vi "PvgeneratorOP300.2.vi"(8 "errin":errorcluster, 10 "network":path, 11 "path in":path) -> (0 "sortie d'erreur":errorcluster caption="errout", 1 "network out":path, 2 "tout bon":bool, 3 "Chaîne":string)   [LabVIEW 2020]
uses:
  VG/IS30%.vi
  VG/PN.vi
  <vilib>/Utility/config.llb/NI_LVConfig.lvlib
  SubVI/VG_HYDRAU.vi
panel:
  out "nombre de remplacements":i32
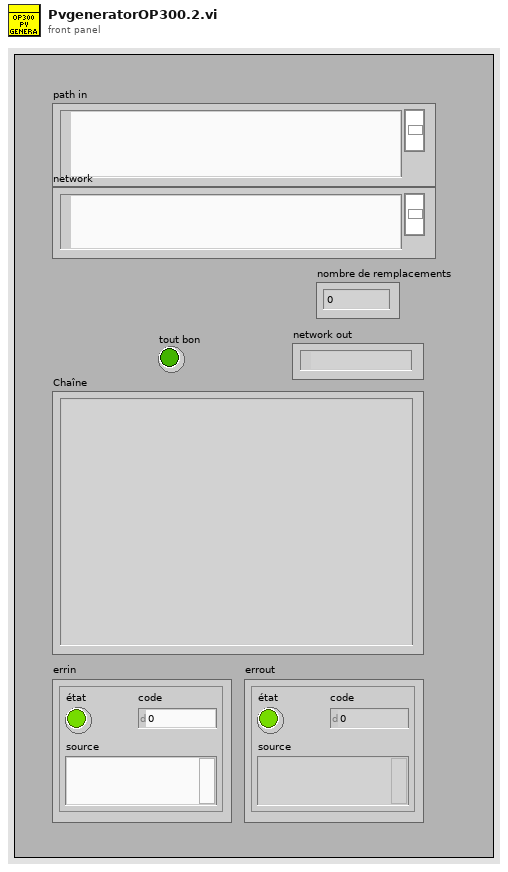
[diagram p1: front panel]
types:
  T1 = enum16{"open", "replace", "create", "open or create", "replace or create", "replace or create with confirmation"}
  T2 = typedef "NI_LVConfig.lvlib/Config Data RefNum.ctl" = refnum<k1>
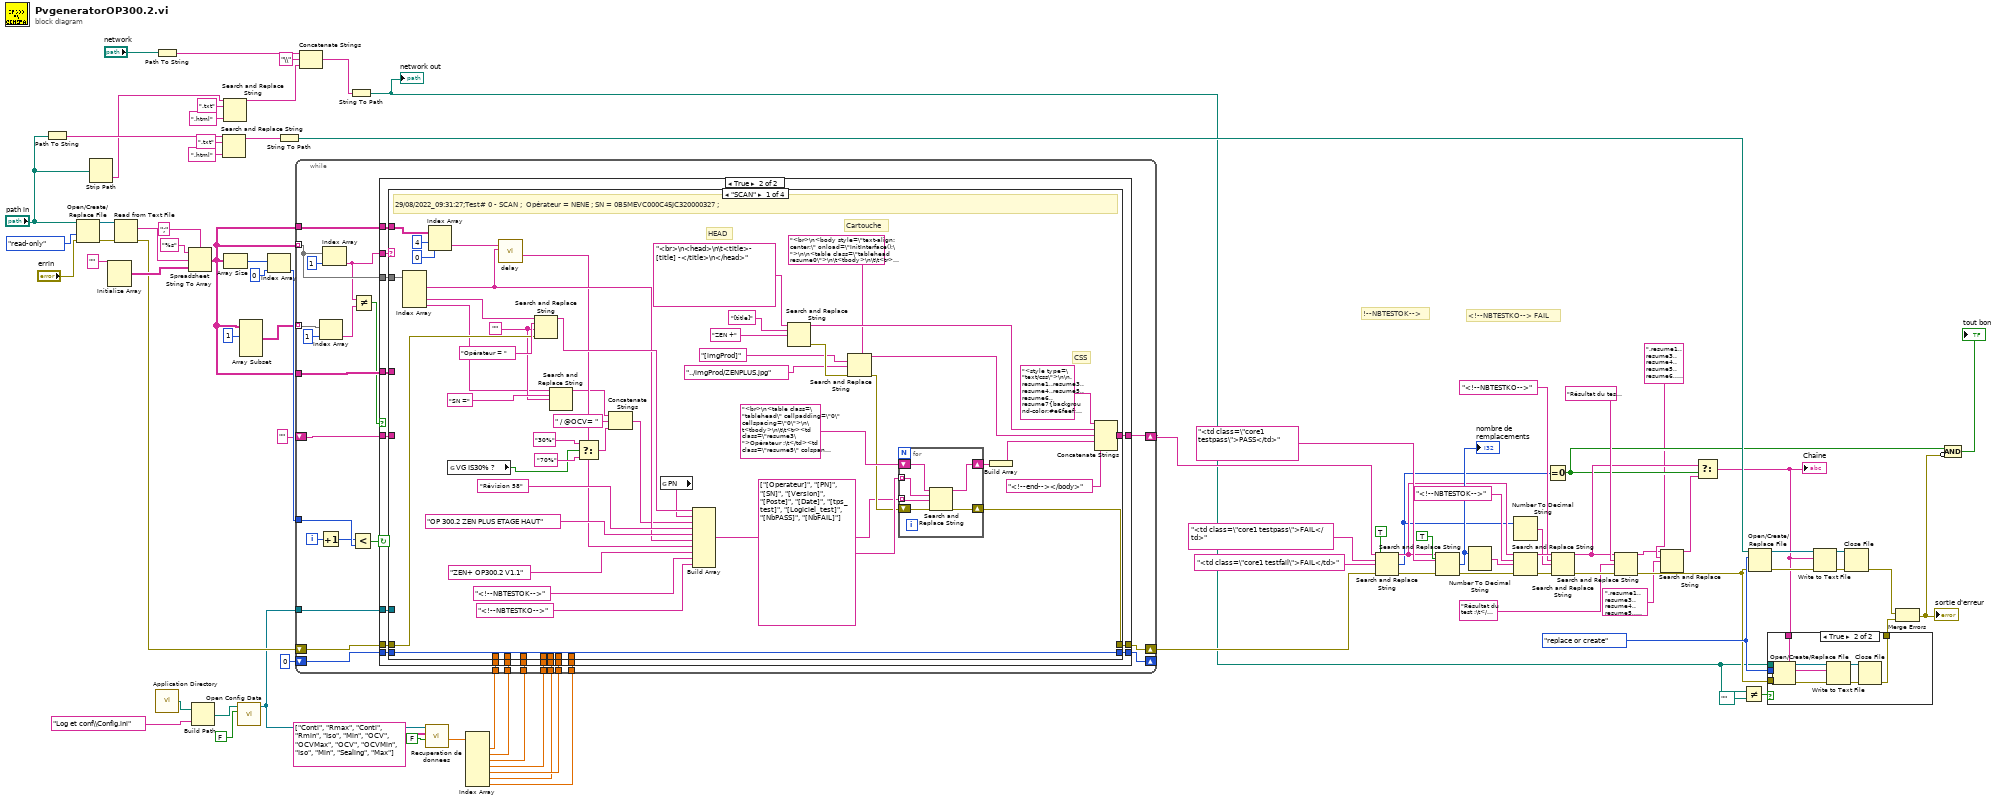
[diagram p0: block diagram]
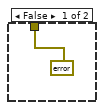
[diagram p2: hidden frame]
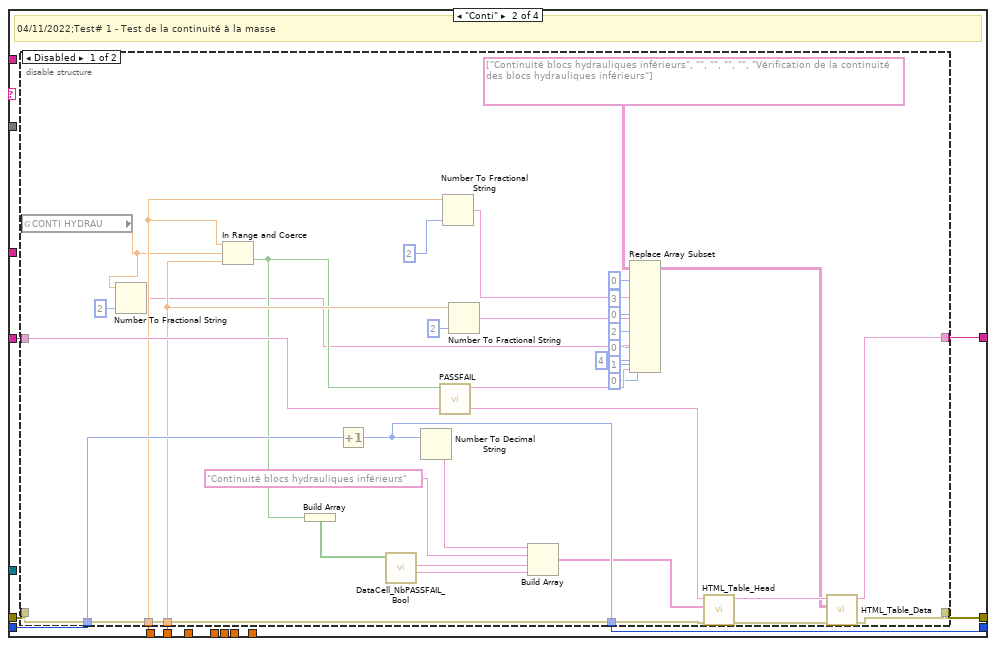
[diagram p4: hidden frame]
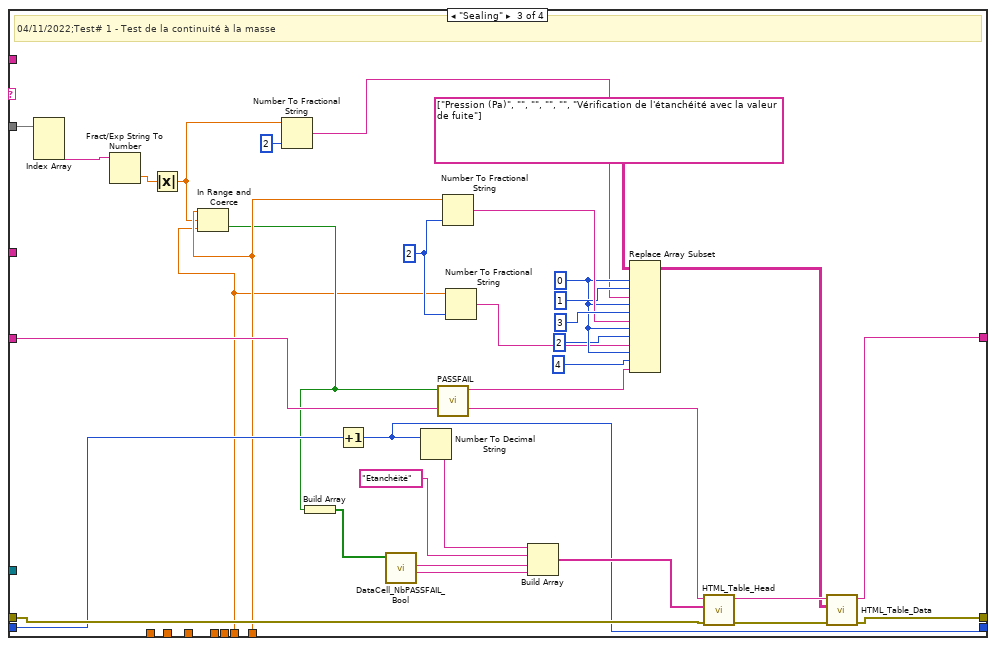
[diagram p6: hidden frame]
diagram:
  w47 = T1."replace or create" ("opération (0 : open)")
  # "<!--NBTESTKO--> FAIL"
  # "!--NBTESTOK-->"
  n1 = Path To String(path="path in") -> (string=w69:string)
  n2 = Open/Create/Replace File(file path (use dialog)="path in", error in="errin", access (0:read/write)=enum16{"read/write", "read-only", "write-only"}."read-only" ("accès (0 : read/write)")) -> (refnum out=w70:refnum<file>, error out=w87:errorcluster)  [unwired: 3 in, 1 out]
  n3 = Strip Path(path="path in") -> (name=w28:string)  [unwired: 1 out]
  n4 = Initialize Array("") -> (w85:string[][])  [unwired: 2 in]
  n5 = Read from Text File(file (use dialog)=w70, error in=w87) -> (text=w83:string, error out=w75:errorcluster)  [unwired: 2 in, 2 out]
  n6 = Path To String(path="network") -> (string=w27:string)
  n7 = call <vilib>:"Application Directory.vi"() -> ("Application Directory"=w19:path)
  n8 = Spreadsheet String To Array(delimiter (Tab)=";" ("séparateur (Tabulation)"), format string="%s" ("chaîne de format"), spreadsheet string=w83, array type (2D Dbl)=w85) -> (array=w6:string[][])
  n9 = Build Path(base path=w19, name or relative path="Log et conf\\Config.ini") -> (appended path=w22:path)
  n10 = Search and Replace String(input string=w69, search string=".txt" ("chaîne recherchée"), replace string=".html" ("chaîne de remplacement (\"\")")) -> (result string=w66:string)  [unwired: 5 in, 3 out]
  n11 = Search and Replace String(input string=w28, search string=".txt" ("chaîne recherchée"), replace string=".html" ("chaîne de remplacement (\"\")")) -> (result string=w25:string)  [unwired: 5 in, 3 out]
  n12 = Array Size(array=w6) -> (size(s)=w81:i32[])
  n13 = call <vilib>:"Open Config Data.vi"("create file if necessary (T)"=FALSE, "configuration file path"=w22) -> ("refnum"=w1:T2)  [unwired: 7 in, 2 out]
  n14 = Array Subset(array=w6, index (row)=1 ("indice")) -> (w4:string[][])  [unwired: 3 in]
  n15 = Index Array(array=w81, index=0 ("indice")) -> (element=w79:i32)
  n16 = String To Path(string=w66) -> (path=w65:path)
  n17 = Concatenate Strings(w27, "\\" ("chaîne"), w25) -> (w24:string)
  n18 = String To Path(string=w24) -> (path=w30:path)
  "network out" <- w30
  n19 = call "Recuperation de donnees.vi"("Est-ce un string?"=FALSE, "Array in"=string[][] [["Conti", "Rmax"], ["Conti", "Rmin"], ["Iso", "Min"], ["OCV", "OCVMax"], ["OCV", "OCVMin"], ["Iso", "Min"], ["Sealing", "Max"]], "Refnum in"=w1) -> ("Array"=w16:dbl[])  [unwired: 7 in, 1 out]
  n20 = Index Array(array=w16) -> (element #1=w15:dbl, element #2=w14:dbl, element #3=w13:dbl, element #4=w12:dbl, element #5=w11:dbl, element #6=w3:dbl, element #7=w2:dbl)  [unwired: 7 in]
  n21 = while {
    tunnel: w79 -> [w114]
    tunnel: w6 -> [w111] mode=indexing
    shift-right: [w110] -> w62
    shift-left: w75 -> [w109]
    shift-right: [w103] -> w64
    shift-left: "" -> [w108]
    shift-right: [w106] -> _
    shift-left: 0 -> [w107]
    tunnel: w6 -> [w105]
    tunnel: w15 -> [w102]
    tunnel: w14 -> [w101]
    tunnel: w6 -> [w100]
    tunnel: w13 -> [w99]
    tunnel: w12 -> [w98]
    tunnel: w11 -> [w97]
    tunnel: w4 -> [w95] mode=indexing
    tunnel: w3 -> [w91]
    tunnel: w2 -> [w90]
    tunnel: w1 -> [w89]
    i -> [w115]
    stop <- w113 continue-if-true
    n22 = Index Array(array=w95, index=1 ("indice")) -> (element=w94:string)
    n23 = Increment(x=w115) -> (x+1=w104:i32)
    n24 = Index Array(array=w111, index=1 ("indice")) -> (element=w93:string)
    n25 = Less?(x=w104, y=w114) -> (x < y?=w113:bool)
    n26 = Not Equal?(x=w93, y=w94) -> (x != y?=w92:bool)
    n27 = case shown="True" w92 {
      tunnel: w111 -> [_ w136]
      tunnel: [w117 w135] -> w110
      tunnel: w109 -> [w117 w134]
      tunnel: w108 -> [w118 w133]
      tunnel: w107 -> [w116 w132]
      tunnel: [w116 w131] -> w106
      tunnel: w105 -> [_ w130]
      tunnel: [w118 w129] -> w103
      tunnel: w93 -> [_ w128]
      tunnel: w102 -> [_ w127]
      tunnel: w101 -> [_ w126]
      tunnel: w100 -> [_ w125]
      tunnel: w99 -> [_ w124]
      tunnel: w98 -> [_ w123]
      tunnel: w97 -> [_ w122]
      tunnel: w91 -> [_ w121]
      tunnel: w90 -> [_ w120]
      tunnel: w89 -> [_ w119]
      frame False {
      }
      frame True {
        n28 = case shown="\"SCAN\"" w128 {
          tunnel: w134 -> [w181 w197 w259 w269]
          tunnel: w136 -> [w183 _ w260 _]
          tunnel: [w160 w196 w258 w269] -> w135
          tunnel: w133 -> [_ w195 w257 w267]
          tunnel: w132 -> [w159 w194 w256 w268]
          tunnel: [w159 w193 w255 w268] -> w131
          tunnel: w130 -> [_ _ _ _]
          tunnel: [w158 w192 w254 w267] -> w129
          tunnel: w127 -> [_ w191 _ _]
          tunnel: w126 -> [_ w190 _ _]
          tunnel: w125 -> [w151 _ _ _]
          tunnel: w124 -> [_ _ _ _]
          tunnel: w123 -> [_ _ _ _]
          tunnel: w122 -> [_ _ w238 _]
          tunnel: w121 -> [_ _ _ _]
          tunnel: w120 -> [_ _ w242 _]
          tunnel: w119 -> [_ _ _ _]
          frame "SCAN" {
            w154 = ""
            # "Cartouche"
            # "HEAD"
            # "CSS"
            # "29/08/2022_09:31:27;Test# 0 - SCAN ;  Opérateur = NENE ; SN = 0B5MEVC000C45JC320000327 ;"
            n29 = Index Array(array=w183) -> (element #1=w147:string, element #3=w157:string, element #4=w152:string)  [unwired: 4 in, 1 out]
            n30 = Index Array(array=w151, index (row)=4, index (col)=0 ("disabled index (col)")) -> (element=w148:string)
            n31 = global read "IS30%.vi" "VG IS30% ?"() -> (w138:bool)
            n32 = call "delay.vi"("String"=w147, "String 2"=w148) -> ("Delay calculé"=w146:string)  [unwired: 9 in]
            n33 = Search and Replace String(input string=w157, search string="Opérateur = " ("chaîne recherchée"), replace string=w154, error in=w181) -> (result string=w156:string)  [unwired: 4 in, 3 out]
            n34 = Search and Replace String(input string=w152, search string="SN =" ("chaîne recherchée"), replace string=w154) -> (result string=w144:string)  [unwired: 5 in, 3 out]
            n35 = Select(t="30%" ("y"), s=w138, f="70%" ("y")) -> (s? t:f=w141:string)
            n36 = Concatenate Strings(w144, " / @OCV= " ("chaîne"), w141) -> (w143:string)
            n37 = global read "PN.vi" "PN"() -> (w137:string)
            n38 = Build Array(w156, w137, w143, "Révision 58" ("element"), "OP 300.2 ZEN PLUS ETAGE HAUT" ("chaîne"), w147, w146, "ZEN+ OP300.2 V1.1" ("chaîne"), "<!--NBTESTOK-->" ("chaîne"), "<!--NBTESTKO-->" ("chaîne")) -> (w161:string[])
            n39 = Search and Replace String(input string="<br>\n<head>\n\t<title>- [title] -</title>\n</head>", search string="[title]" ("chaîne recherchée"), replace string="ZEN +" ("Title")) -> (result string=w177:string, error out=w176:errorcluster)  [unwired: 5 in, 2 out]
            n40 = Search and Replace String(input string="<br>\n<body style=\"text-align: center;\" onload=\"InitInterface();\">\n\n<table class=\"tablehead resume0\">\n\t<tbody>\n\t\t<tr>\n\t\t\t<td> <img src=\"[imgProd]\" style=\"width:194px;height:100px\" class=\"left\"></td>\n\t\t\t<td> <div class=\"center\">PROCES VERBAL DE TEST AUTOMATIQUE</div><div class=\"center\">Zen Plus OP 300.2</div><br class=\"center\"><div class=\"center\">Forseepower</div></td>\n\t\t\t<td> <img src=\"../imgProd/LOGO FORSEE.png\" style=\"width:auto;height:auto\"  class=\"right\"></td>\n\t\t</tr>\n\t</tbody>\n</table>", search string="[imgProd]", replace string="../imgProd/ZENPLUS.jpg" ("imgProd"), error in=w176) -> (result string=w174:string, error out=w171:errorcluster)  [unwired: 4 in, 2 out]
            n41 = for {
              shift-right: [w188] -> w170
              shift-left: "<br>\n<table class=\"tablehead\" cellpadding=\"0\" cellspacing=\"0\">\n\t<tbody>\n\t\t<tr><td class=\"resume3\">Opérateur :\t</td><td class=\"resume5\" colspan=\"3\">[Operateur]</td></tr>\n\t\t<tr><td class=\"resume3\">PN : </td><td class=\"resume5\" colspan=\"3\">[PN]</td></tr>\n\t\t<tr><td class=\"resume3\">SN : </td><td class=\"resume5\" colspan=\"3\">[SN]</td></tr>\n\t\t<tr><td class=\"resume3\">Version : </td><td class=\"resume5\" colspan=\"3\">[Version]</td></tr>\n\t\t<tr><td class=\"resume3\">Poste : </td><td class=\"resume5\" colspan=\"3\">[Poste]</td></tr>\t\t\n\t\t<tr><td class=\"resume3\">Date du test : </td><td class=\"resume5\" colspan=\"3\">[Date]</td></tr>\n\t\t<tr><td class=\"resume3\">Temps de test : </td><td class=\"resume5\" colspan=\"3\">[tps_test]</td></tr>\n\t\t<tr><td class=\"resume3\">Logiciel de test :\t</td><td class=\"resume5\" colspan=\"3\">[Logiciel_test]</td></tr>\n\t\t<tr><td class=\"resume3\">Résultat du test :\t</td><td class=\"resume5\" colspan=\"3\"><div><span style=\"float:left\" id=\"result\"><font size = \"5pt\" color=\"green\"><b>CONFORME</b></font><b><font size = \"5pt\"> ( </font><font size = \"5pt\" color=\"green\">[NbPASS] PASS </font>  <font size = \"5pt\"> / </font><font size = \"5pt\" color=\"red\">[NbFAIL] FAIL</font> <font size = \"5pt\"> ) </font></b></span></div></td></tr>\n\t</tbody>\n</table>" -> [w189]
              tunnel: string[] ["[Operateur]", "[PN]", "[SN]", "[Version]", "[Poste]", "[Date]", "[tps_test]", "[Logiciel_test]", "[NbPASS]", "[NbFAIL]"] -> [w185] mode=indexing
              tunnel: w161 -> [w184] mode=indexing
              shift-right: [w186] -> w160
              shift-left: w171 -> [w187]
              n42 = Search and Replace String(input string=w189, search string=w185, replace string=w184, error in=w187) -> (result string=w188:string, error out=w186:errorcluster)  [unwired: 4 in, 2 out]
            }
            n43 = Build Array(w170) -> (w169:string[])
            n44 = Concatenate Strings("<style type=\"text/css\">\n\n.resume1,.resume3,.resume4,.resume5,.resume6,.resume7{background-color:#e6feef;padding:7px;border:1px solid black;}\n.resume0{border:1px solid black;background-color:#e6feef;font-weight: bold;padding:0px;text-align: center;}\n.resume1{width:350px;text-align:right;font-weight:bold;}\n.resume3{width:350px;text-align:right;border-top:0px solid black;font-weight:bold;}\n.resume4{border-left:0px solid black;width:290px;}\n.resume5{width:290px;border-left:0px solid black;border-top:0px solid black;}\n.resume6{border-left:0px solid black;width:60px;}\n.resume7{border-left:0px solid black;border-top:0px solid black;width:60px;}\n.title1{text-align: left;background-color:#e6f4fe;padding:10px;border:1px solid #101010;}\n.title2{width: 30px;text-align: center;background-color:#e6f4fe;padding:1px;border:1px solid #101010;border-left:0px solid black;font-weight: bold;}\n.title2 a:link{text-decoration:none;}\n.entete0,.entete1,.entete2,.time2{text-align: center;background-color:#feeec9;padding:7px;border:1px solid black;font-weight: bold;}\n.entete0{width:45px;border-right:0px solid black;}\n.entete1{width:505px;}\n.entete2{width:95px;border-right:0px solid black;}\n.time2{border-left:0px solid black;width:145px;font-size:11px;}\n.core0,.core1,.core2,.core3,.core4,.time{text-align: center;background-color:#fafed3;padding:7px;border:1px solid black;}\n.core0, .core1,.core3,.core4{width:95px;border-top:0px solid black;border-right:0px solid black;}\n.core0{width:45px;}\n.core2{border-top:0px solid black;width:505px;}\n.core3{width:200px;}\n.core4{width:300px;}\n.time{width:145px;border-top:0px solid black;border-left:0px solid black;font-size:11px;}\n.false .core0,.false .core1,.false .core2,.false .core3,.false .core4,.false .time{background-color:#f4f4f4;}\n.false .entete0,.false .entete1,.false .entete2,.false .time2{background-color:#dadada;}\n.false .title1,.false .title2,.false .resultentete .testpass,.false .resultentete .testfail,.false .resultentete .testtime{background-color:#c5cac9;color: blue;}\n.false .title2 a:link{text-decoration:none;color: blue;}\n.comment1,.comment2,.time3{width: 890px;background-color:#e9e8e9;padding:7px;border:1px solid black;border-top:0px solid black;text-align:left;}\n.comment2{border-right:0px solid black;width: 45px;text-align: center;}\n.time3{width: 145px;border-left:0px solid black;font-size:11px;}\n.fixe1{background: -moz-linear-gradient(center top , #101010 10%, #555555 80%) repeat scroll 0 0 transparent;background: -webkit-gradient(linear, left top, left bottom, from(#101010), to(#555555));border:2px solid orange;position : fixed;margin-top:20px;display:none;overflow-y:scroll;max-height:350px;text-shadow: 0px 0px 0 #333333;text-align:left;font-size:10px;padding:10px;margin-left:-162px;border-radius: 15px 15px 15px 15px;}\n.menufixe, .menufixelock{background: -moz-linear-gradient(center top , #101010 80%, transparent 20%) repeat scroll 0 0 transparent;background: -webkit-gradient(linear, left top, left bottom, from(#101010), color-stop(0.65, #101010), to(transparent)) repeat scroll 0 0 transparent;margin: -52px 0px 0px -9px;width:100%;position:fixed;height:55px;-moz-transition: margin 1s;-webkit-transition: margin 1s;}\n.menufixelock, .menufixe:hover{margin: -9px 0px 0px -9px;}\n.lockmenu, .separation,.separationmenu{text-align:center;background: -moz-linear-gradient(center top , #555555 10%, #111111 80%) repeat scroll 0 0 transparent;background: -webkit-gradient(linear, left top, left bottom, from(#555555), to(#111111));border: 1px solid white;border-radius: 10px 10px 10px 10px;box-shadow: 0 -1px 1px #555555 inset;color: #999999;font-weight: bold;width: 100px;padding: 2px;text-decoration: none;}\n.tablehead{width: 1000px;font-family: Verdana;font-size: 12px;margin-left: auto;margin-right: auto;}\n.tablenull{font-family: Verdana;font-size: 11px;margin-left: auto;margin-right: auto;}\n.separationmenu:hover div{display: inline;}\n.lockmenu:hover, .separation:hover,.separationmenu:hover{border: 1px solid orange;cursor:pointer;}\n.lockmenu:hover{border: 1px solid red;cursor:pointer;}\n.separationright{padding:10px;}\ndiv a:link{text-decoration:none;color:#cbcbcb;}\ndiv a:hover{text-decoration:underline;color:#cbcbcb;}\nspan a:link{text-decoration:none;color:#cbcbcb;}\nspan a:hover{text-decoration:none;color:#cbcbcb;}\n.false{color: blue;}\n.testpass{color: green;font-weight: bold;}\n.testfail{color: red;font-weight: bold;}\n.testtime{color: blue;font-weight: bold;}\n.resultentete{font-weight: bold;font-size: 11px;min-width: 200px;text-align:right;}\n.infohard{border: 1px solid black;background-color: white;text-align: center;width: 16px;height: 16px;border-radius: 5px;font-weight: bold;box-shadow: 0 -1px 2px #555555 inset;}\n.infohard:hover{background-color:#feeec9;cursor:pointer;}\n.footerhard{padding-top:30px;}\n.confighard{font-size:10px;width:110px;}\n.circlemain{margin-left:auto;margin-right:auto;}\n.circletext,.circleform{padding-top: 3px;text-align:center;font-size: 10px;width:200px;}\n.circleform{padding-bottom: 3px;padding-top: 1px;}\n.circle{border: 1px solid black;border-collapse: collapse;border-radius: 15px;box-shadow: 1px 1px 0 #505050;height: 15px;width: 15px;display:inline-block;}\n.bookmarkon, .bookmarkoff{background-color: yellow;border: 1px solid black;border-collapse: collapse;border-radius: 10px 10px 10px 10px;box-shadow: 1px 1px 0 #505050;height: 12px;width: 12px;position: absolute;margin-left:22px;cursor: help;}\n.bookmarkoff{background-color: transparent;border: 1px solid #CECECE;box-shadow: none;cursor: copy;}\n.false .bookmarkoff{background-color: transparent;border: 1px solid #E6E1E1;box-shadow: none;cursor: copy;}\n.bookmarkmaster{height: 15px;margin-right: 12px;width: 60px;}\n.bookmarkmaster:hover .bookmarkprev,.bookmarkmaster:hover .bookmarksuiv{display:block;}\n.bookmarkprev, .bookmarksuiv {cursor: pointer;font-size: 25px;font-weight: bold;margin-top: -10px;position: absolute;display:none;}\n.bookmarkprev{margin-left: 2px;}\n.bookmarksuiv{margin-left: 43px;}\n.plus, .moins{background-color: #F4F4F4;border: 1px solid #848484;border-radius: 20px;color: #848484;font-family: arial;font-size: 16px;font-weight: bold;height: 20px;margin-left: 4px;text-align: center;width: 20px;}\n.moins{font-size: 15px;}\n.plus:hover, .moins:hover{background-color: #DADADA;border: 1px solid black;color: black;cursor:pointer;}\n.backtothetop {position: fixed; right: 50%; margin-right: -555px; bottom: 10px; font-size: 35px; font-weight: bold; border: 1px solid #7D7B91; width: 40px; height: 40px; line-height:52px; text-align: center;border-radius: 8px; opacity: 0.25; background-color: #F5F5F5; color:#7D7B91;}\n.backtothetop:hover {opacity: 1; cursor:pointer;}\n.libversion {font-size: 8px;font-weight: normal;padding-right: 10px;text-align: right;}\n.lockmenu {width: 18px;font-size: 12px;}\n.left {display: block; margin-left: 1px;margin-right: auto;}\n.right {display: block; margin-right: 1px;margin-left: auto;}\n.center {display: block; margin-left: auto;margin-right: auto;}\n\n</style>", w177, w174, w169, "<!--end--></body>") -> (w158:string)
          }
          frame "Conti" {
            # "04/11/2022;Test# 1 - Test de la continuité à la masse"
            n45 = disable-structure shown="Disabled" {
              disable-tunnel: w197 -> [w232 _]
              disable-tunnel: [w231 _] -> w196
              disable-tunnel: w195 -> [w230 _]
              disable-tunnel: w194 -> [w229 _]
              disable-tunnel: [w228 _] -> w193
              disable-tunnel: [w227 _] -> w192
              disable-tunnel: w191 -> [w226 _]
              disable-tunnel: w190 -> [w225 _]
              frame Disabled {
                n46 = global read "VG_HYDRAU.vi" "CONTI HYDRAU"() -> (w211:dbl)
                n47 = Number To Fractional String(number=w211, precision (6)=i16 2 ("précision (6)")) -> (F-format string=w203:string)  [unwired: 2 in]
                n48 = In Range and Coerce(upper limit=w226, x=w211, lower limit=w225) -> (In Range?=w212:bool)  [unwired: 1 out]
                n49 = Build Array(w212) -> (w217:bool[])
                n50 = Increment(x=w229) -> (x+1=w228:i32)
                n51 = call "DataCell_NbPASSFAIL_Bool.vi"("Tableau en entrée"=w217) -> ("Chaîne"=w215:string, "Chaîne 2"=w216:string)  [unwired: 8 in, 1 out]
                n52 = Number To Decimal String(number=w228) -> (decimal integer string=w220:string)  [unwired: 1 in]
                n53 = call <userlib>:"PASSFAIL.vi"("E"=w212) -> ("S"=w200:string)  [unwired: 10 in]
                n54 = Number To Fractional String(number=w226, precision (6)=i16 2) -> (F-format string=w209:string)  [unwired: 2 in]
                n55 = Number To Fractional String(number=w225, precision (6)=i16 2) -> (F-format string=w206:string)  [unwired: 2 in]
                n56 = Build Array(w220, "Continuité blocs hydrauliques inférieurs" ("élément"), w216, w215) -> (w223:string[])
                n57 = Replace Array Subset(array=string[][] [["Continuité blocs hydrauliques inférieurs", "", "", "", "", "Vérification de la continuité des blocs hydrauliques inférieurs"]] ("Tableau"), new element #1=w209, index (row) #1=0 ("indice (ligne)"), index (col) #1=3 ("indice désactivé (col)"), new element #2=w206, index (row) #2=0 ("indice (ligne)"), index (col) #2=2 ("indice désactivé (col)"), new element #3=w203, index (row) #3=0 ("indice (ligne)"), index (col) #3=1 ("indice désactivé (col)"), new element #4=w200, index (row) #4=0 ("indice (ligne)"), index (col) #4=4 ("indice désactivé (col)")) -> (w218:string[][])
                n58 = call "HTML_Table_Head.vi"("entrée d'erreur (pas d'erreur)"=w232, "Tableau"=w223, "chaîne en entrée"=w230) -> ("sortie d'erreur"=w222:errorcluster, "result string"=w221:string)  [unwired: 7 in]
                n59 = call "HTML_Table_Data.vi"("entrée d'erreur (pas d'erreur)"=w222, "Tableau"=w218, "chaîne en entrée"=w221) -> ("sortie d'erreur"=w231:errorcluster, "result string"=w227:string)  [unwired: 7 in]
              }
              frame Enabled {
              }
            }
          }
          frame "Sealing" {
            w239 = i16 2 ("precision (6)")
            w244 = 0 ("index (row)")
            # "04/11/2022;Test# 1 - Test de la continuité à la masse"
            n60 = Index Array(array=w260) -> (element #3=w247:string)  [unwired: 3 in, 2 out]
            n61 = Fract/Exp String To Number(string=w247) -> (number=w236:dbl)  [unwired: 3 in, 1 out]
            n62 = Absolute Value(x=w236) -> (abs(x)=w235:dbl)
            n63 = In Range and Coerce(upper limit=w242, x=w235, lower limit=w238) -> (In Range?=w241:bool)  [unwired: 1 out]
            n64 = Number To Fractional String(number=w235, precision (6)=i16 2 ("précision (6)")) -> (F-format string=w234:string)  [unwired: 2 in]
            n65 = Build Array(w241) -> (w240:bool[])
            n66 = Increment(x=w256) -> (x+1=w255:i32)
            n67 = call "DataCell_NbPASSFAIL_Bool.vi"("Tableau en entrée"=w240) -> ("Chaîne"=w251:string, "Chaîne 2"=w252:string)  [unwired: 8 in, 1 out]
            n68 = Number To Decimal String(number=w255) -> (decimal integer string=w262:string)  [unwired: 1 in]
            n69 = call <userlib>:"PASSFAIL.vi"("E"=w241) -> ("S"=w246:string)  [unwired: 10 in]
            n70 = Number To Fractional String(number=w242, precision (6)=w239) -> (F-format string=w249:string)  [unwired: 2 in]
            n71 = Number To Fractional String(number=w238, precision (6)=w239) -> (F-format string=w237:string)  [unwired: 2 in]
            n72 = Build Array(w262, "Etanchéité" ("élément"), w252, w251) -> (w265:string[])
            n73 = Replace Array Subset(array=string[][] [["Pression (Pa)", "", "", "", "", "Vérification de l'étanchéité avec la valeur de fuite"]] ("Tableau"), new element #1=w234, index (row) #1=w244, index (col) #1=1 ("disabled index (col)"), new element #2=w249, index (row) #2=w244, index (col) #2=3 ("disabled index (col)"), new element #3=w237, index (row) #3=w244, index (col) #3=2 ("disabled index (col)"), new element #4=w246, index (row) #4=w244, index (col) #4=4 ("disabled index (col)")) -> (w253:string[][])
            n74 = call "HTML_Table_Head.vi"("entrée d'erreur (pas d'erreur)"=w259, "Tableau"=w265, "chaîne en entrée"=w257) -> ("sortie d'erreur"=w264:errorcluster, "result string"=w263:string)  [unwired: 7 in]
            n75 = call "HTML_Table_Data.vi"("entrée d'erreur (pas d'erreur)"=w264, "Tableau"=w253, "chaîne en entrée"=w263) -> ("sortie d'erreur"=w258:errorcluster, "result string"=w254:string)  [unwired: 7 in]
          }
          frame "NULL", Default {
            # "NULL"
          }
        }
      }
    }
  }
  n76 = Search and Replace String(replace all?=TRUE ("tout remplacer ? (F)"), input string=w64, search string="<td class=\"core1 testpass\">FAIL</td>" ("chaîne recherchée"), replace string="<td class=\"core1 testfail\">FAIL</td>" ("chaîne de remplacement (\"\")"), error in=w62) -> (result string=w48:string, number of replacements=w43:i32, error out=w59:errorcluster)  [unwired: 3 in, 1 out]
  n77 = Search and Replace String(replace all?=TRUE ("tout remplacer ? (F)"), input string=w48, search string="<td class=\"core1 testpass\">PASS</td>" ("chaîne recherchée"), error in=w59) -> (number of replacements=w51:i32, error out=w55:errorcluster)  [unwired: 4 in, 2 out]
  "nombre de remplacements" <- w51
  n78 = Number To Decimal String(number=w51) -> (decimal integer string=w50:string)  [unwired: 1 in]
  n79 = Number To Decimal String(number=w43) -> (decimal integer string=w49:string)  [unwired: 1 in]
  n80 = Search and Replace String(input string=w48, search string="<!--NBTESTOK-->" ("chaîne recherchée"), replace string=w50, error in=w55) -> (result string=w56:string, error out=w54:errorcluster)  [unwired: 4 in, 2 out]
  n81 = Equal To 0?(x=w43) -> (x = 0?=w35:bool)
  n82 = Search and Replace String(input string=w56, search string="<!--NBTESTKO-->" ("chaîne recherchée"), replace string=w49, error in=w54) -> (result string=w38:string, error out=w42:errorcluster)  [unwired: 4 in, 2 out]
  n83 = Search and Replace String(input string=w38, search string="Résultat du test :\t</td><td class=\"resume5\" colspan=\"3\"><div><span style=\"float:left\" id=\"result\"><font size = \"5pt\" color=\"green\"><b>CONFORME</b>", replace string="Résultat du test :\t</td><td class=\"resume5\" colspan=\"3\"><div><span style=\"float:left\" id=\"result\"><font  size = \"5pt\" color=\"red\"><b>NON CONFORME</b>", error in=w42) -> (result string=w8:string, error out=w41:errorcluster)  [unwired: 4 in, 2 out]
  n84 = Search and Replace String(input string=w8, search string=".resume1,.resume3,.resume4,.resume5,.resume6,.resume7{background-color:#e6feef;padding:7px;border:1px solid black;}\n.resume0{border:1px solid black;background-color:#e6feef;font-weight: bold;padding:0px;text-align: center;}", replace string=".resume1,.resume3,.resume4,.resume5,.resume6,.resume7{background-color:#fdebd0;padding:7px;border:1px solid black;}\n.resume0{border:1px solid black;background-color:#fdebd0;font-weight: bold;padding:0px;text-align: center;}") -> (result string=w7:string)  [unwired: 5 in, 3 out]
  n85 = Select(t=w38, s=w35, f=w7) -> (s? t:f=w39:string)
  "Chaîne" <- w39
  n86 = Not Equal?(x=w30, y=path "") -> (x != y?=w32:bool)
  n87 = Open/Create/Replace File(file path (use dialog)=w65, error in=w41, operation (0:open)=w47) -> (refnum out=w71:refnum<file>, error out=w73:errorcluster)  [unwired: 3 in, 1 out]
  n88 = case shown="True" w32 {
    tunnel: w47 -> [_ w275]
    tunnel: w30 -> [_ w274]
    tunnel: w41 -> [_ w273]
    tunnel: w39 -> [_ w272]
    tunnel: [errorcluster {"status"=FALSE, "code"=0, "source"=""} ("error out") w271] -> w37
    frame False {
    }
    frame True {
      n89 = Open/Create/Replace File(file path (use dialog)=w274, error in=w273, operation (0:open)=w275) -> (refnum out=w276:refnum<file>, error out=w278:errorcluster)  [unwired: 3 in, 1 out]
      n90 = Write to Text File(file (use dialog)=w276, text=w272, error in=w278) -> (refnum out=w277:refnum<file>, error out=w279:errorcluster)  [unwired: 1 in, 1 out]
      n91 = Close File(refnum=w277, error in=w279) -> (error out=w271:errorcluster)  [unwired: 1 out]
    }
  }
  n92 = Write to Text File(file (use dialog)=w71, text=w39, error in=w73) -> (refnum out=w72:refnum<file>, error out=w74:errorcluster)  [unwired: 1 in, 1 out]
  n93 = Close File(refnum=w72, error in=w74) -> (error out=w36:errorcluster)  [unwired: 1 out]
  n94 = Merge Errors(w36, w37) -> (w34:errorcluster)
  "sortie d'erreur" <- w34
  n95 = Compound Arithmetic op=AND ("Opérateur arithmétique")(w35, invert w34) -> (→"tout bon":bool)
